vi "Utility Create INI Path.vi"(11 "VI Ref In":refnum<vi>) -> (3 "INI Path":path)   [LabVIEW 2020]
panel:
  out "error out":errorcluster
  in  "error in (no error)":errorcluster
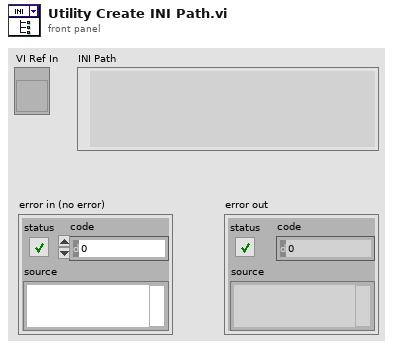
[diagram p1: front panel]
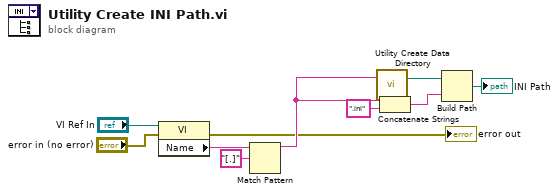
[diagram p0: block diagram]
diagram:
  n1 = property class="VI"(reference="VI Ref In", error in="error in (no error)") -> (error out=→"error out":errorcluster, "Name"=w9:string)  [unwired: 1 out]
  n2 = Match Pattern(string=w9, regular expression="[.]" ("search string")) -> (before substring=w4:string)  [unwired: 1 in, 3 out]
  n3 = call "Utility Create Data Directory.vi"("Folder Name"=w4) -> ("Path"=w5:path)  [unwired: 2 in]
  n4 = Concatenate Strings(w4, ".ini" ("string")) -> (w2:string)
  n5 = Build Path(base path=w5, name or relative path=w2) -> (appended path=→"INI Path":path)
